vi "Elevator Config.vi"(8 "error in (no error)":errorcluster, 11 "Config in":refnum<class "Config.lvclass">) -> (0 "error out":errorcluster, 1 "IDs found?":bool, 2 "Elevator Data":T1={"Wrist"=0, "Left Master"=0, "Left Slave"=0, "Right Master"=0, "Right Slave"=0, "Elevator Wrist PID"={"P"=0.0, "I"=0.0, "D"=0.0, "F"=0.0, "integralZone"=0.0, "allowableClosedLoopError"=0, "maxIntegralAccumulator"=0.0, "closedLoopPeakOutput"=1.0, "closedLoopPeriod"=1}, "Elevator Arm PID"={"P"=0.0, "I"=0.0, "D"=0.0, "F"=0.0, "integralZone"=0.0, "allowableClosedLoopError"=0, "maxIntegralAccumulator"=0.0, "closedLoopPeakOutput"=1.0, "closedLoopPeriod"=1}, "Vacumm Pump 1"=0, "Vacumm Pump 2"=0, "Arm Motion Magic Max Velocity"=0, "Arm Motion Magic Max Acceleration"=0, "Wrist Motion Magic Max Velocity"=0, "Wrist Motion Magic Max Acceleration"=0}, 3 "Config out":refnum<class "Config.lvclass">, 4 "PIDFs found":bool, 5 "File Found?":bool)   [LabVIEW 2018, in "Config.lvlib" / "Config.lvclass"]
doc: "Use this VI to get the configuration for the Elevator CAN IDs"
uses:
  Config.lvclass
  Controls/Elevator Data.ctl
  <vilib>/Rock Robotics/WPI/ThirdParty/Phoenix-LabVIEW/Motor Controller/Controls/CTRE_Phoenix_MotorControl_SlotStructure.ctl
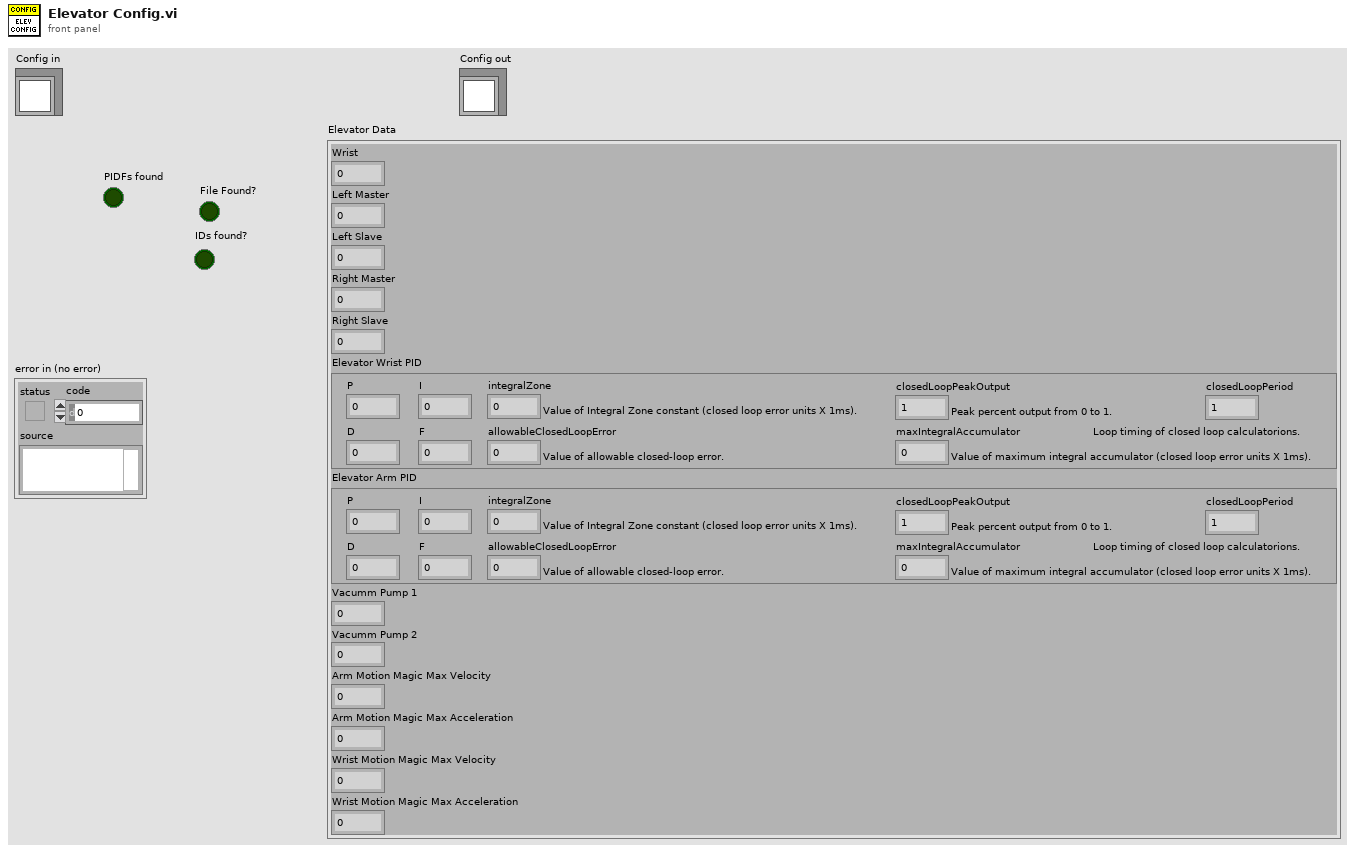
[diagram p1: front panel]
types:
  T1 = typedef "Config.lvlib/Config.lvclass/Elevator Data.ctl" = cluster{"Wrist":u8, "Left Master":u8, "Left Slave":u8, "Right Master":u8, "Right Slave":u8, "Elevator Wrist PID":T2, "Elevator Arm PID":T2, "Vacumm Pump 1":u8, "Vacumm Pump 2":u8, "Arm Motion Magic Max Velocity":u32, "Arm Motion Magic Max Acceleration":u32, "Wrist Motion Magic Max Velocity":u32, "Wrist Motion Magic Max Acceleration":u32}
  T2 = typedef "CTRE_Phoenix_MotorControl_SlotStructure.ctl" = cluster{"P":dbl, "I":dbl, "D":dbl, "F":dbl, "integralZone":dbl, "allowableClosedLoopError":i32, "maxIntegralAccumulator":dbl, "closedLoopPeakOutput":dbl, "closedLoopPeriod":i32}
  T3 = typedef "Config.lvlib/Config.lvclass/Elevator Data.ctl" = cluster{"Wrist":u8, "Left Master":u8, "Left Slave":u8, "Right Master":u8, "Right Slave":u8, "Elevator Wrist PID":T2, "Elevator Arm PID":T2, "Vacumm Pump 1":u8, "Vacumm Pump 2":u8, "Arm Motion Magic Max Velocity":u32, "Arm Motion Magic Max Acceleration":u32, "Wrist Motion Magic Max Velocity":u32, "Wrist Motion Magic Max Acceleration":u32, "Arm Gear Ratio":dbl, "Wrist Gear Ratio":dbl, "C0 Arm":dbl, "C1 Arm":dbl, "C2 Arm":dbl, "H1 Arm":dbl, "H2 Arm":dbl, "C0 Wrist":dbl, "C1 Wrist ":dbl, "C2 Wrist":dbl, "H1 Wrist":dbl, "H2 Wrist":dbl, "Deploy Arm":dbl, "Deploy Wrist":dbl, "Climb Arm":dbl, "Climb Wrist":dbl, "Arm Encoder ABS Value":i32, "Wrist Encoder ABS Value":i32}
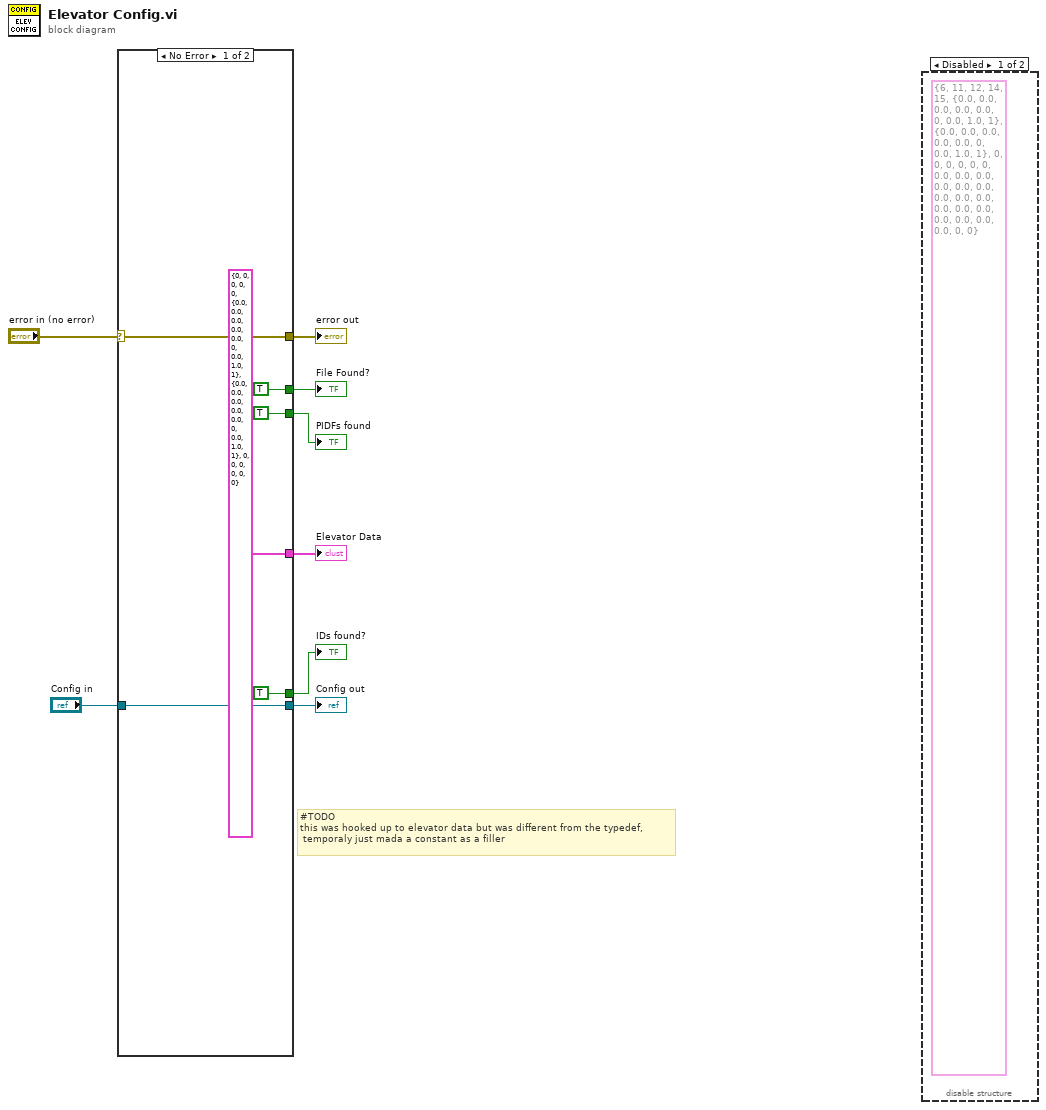
[diagram p0: block diagram]
diagram:
  # "#TODO\nthis was hooked up to elevator data but was different from the typedef,\n temporaly just mada a constant as a filler"
  n1 = case shown="No Error" "error in (no error)" {
    selector: "error in (no error)" -> [w13 w16]
    tunnel: [w13 w16] -> w7
    tunnel: [w14 w15] -> w5
    tunnel: "Config in" -> [w14 w15]
    tunnel: [TRUE ("File Found?") _] -> w4
    tunnel: [TRUE ("IDs found?") _] -> w3
    tunnel: [T1 {"Wrist"=0, "Left Master"=0, "Left Slave"=0, "Right Master"=0, "Right Slave"=0, "Elevator Wrist PID"={"P"=0.0, "I"=0.0, "D"=0.0, "F"=0.0, "integralZone"=0.0, "allowableClosedLoopError"=0, "maxIntegralAccumulator"=0.0, "closedLoopPeakOutput"=1.0, "closedLoopPeriod"=1}, "Elevator Arm PID"={"P"=0.0, "I"=0.0, "D"=0.0, "F"=0.0, "integralZone"=0.0, "allowableClosedLoopError"=0, "maxIntegralAccumulator"=0.0, "closedLoopPeakOutput"=1.0, "closedLoopPeriod"=1}, "Vacumm Pump 1"=0, "Vacumm Pump 2"=0, "Arm Motion Magic Max Velocity"=0, "Arm Motion Magic Max Acceleration"=0, "Wrist Motion Magic Max Velocity"=0, "Wrist Motion Magic Max Acceleration"=0} ("Elevator Data") _] -> w2
    tunnel: [TRUE ("PIDFs found") _] -> w1
    frame No Error {
    }
    frame Error {
    }
  }
  "error out" <- w7
  "Config out" <- w5
  "File Found?" <- w4
  "IDs found?" <- w3
  "Elevator Data" <- w2
  "PIDFs found" <- w1
  n2 = disable-structure shown="Disabled" {
    frame Disabled {
      (unwired) T3 {"Wrist"=6, "Left Master"=11, "Left Slave"=12, "Right Master"=14, "Right Slave"=15, "Elevator Wrist PID"={"P"=0.0, "I"=0.0, "D"=0.0, "F"=0.0, "integralZone"=0.0, "allowableClosedLoopError"=0, "maxIntegralAccumulator"=0.0, "closedLoopPeakOutput"=1.0, "closedLoopPeriod"=1}, "Elevator Arm PID"={"P"=0.0, "I"=0.0, "D"=0.0, "F"=0.0, "integralZone"=0.0, "allowableClosedLoopError"=0, "maxIntegralAccumulator"=0.0, "closedLoopPeakOutput"=1.0, "closedLoopPeriod"=1}, "Vacumm Pump 1"=0, "Vacumm Pump 2"=0, "Arm Motion Magic Max Velocity"=0, "Arm Motion Magic Max Acceleration"=0, "Wrist Motion Magic Max Velocity"=0, "Wrist Motion Magic Max Acceleration"=0, "Arm Gear Ratio"=0.0, "Wrist Gear Ratio"=0.0, "C0 Arm"=0.0, "C1 Arm"=0.0, "C2 Arm"=0.0, "H1 Arm"=0.0, "H2 Arm"=0.0, "C0 Wrist"=0.0, "C1 Wrist "=0.0, "C2 Wrist"=0.0, "H1 Wrist"=0.0, "H2 Wrist"=0.0, "Deploy Arm"=0.0, "Deploy Wrist"=0.0, "Climb Arm"=0.0, "Climb Wrist"=0.0, "Arm Encoder ABS Value"=0, "Wrist Encoder ABS Value"=0} ("Elevator Data")
    }
    frame Enabled {
    }
  }
